vi "SubSubVI.vi"(11 "dataflow in":bool) -> ()   [LabVIEW 2018]
uses:
  98bd6abf-091e-4652-8858-754d125a5b27.vi
  98bd6abf-091e-4652-8858-754d125a5b27.vi/caf2d4a3-5a7b-40e1-b7b0-74b52901b9f9.vi
  98bd6abf-091e-4652-8858-754d125a5b27.vi/caf2d4a3-5a7b-40e1-b7b0-74b52901b9f9.vi/0a1ee2ab-da6d-4243-8cf3-8125e611a602.vi
  api/Log.vi
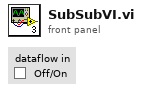
[diagram p1: front panel]
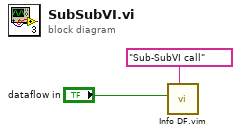
[diagram p0: block diagram]
diagram:
  n1 = call "Info DF.vim"("message"="Sub-SubVI call", "dataflow in"="dataflow in") -> ()  [unwired: 9 in, 1 out]
